vi "GoDef.vi"(8 "error in (no error)":errorcluster, 10 "String 2":string, 11 "Device in":refnum<class "Device.lvclass">) -> (0 "error out":errorcluster, 2 "String":string, 3 "Device out":refnum<class "Device.lvclass">)   [LabVIEW 2018, in "Device.lvclass"]
uses:
  Device.lvclass
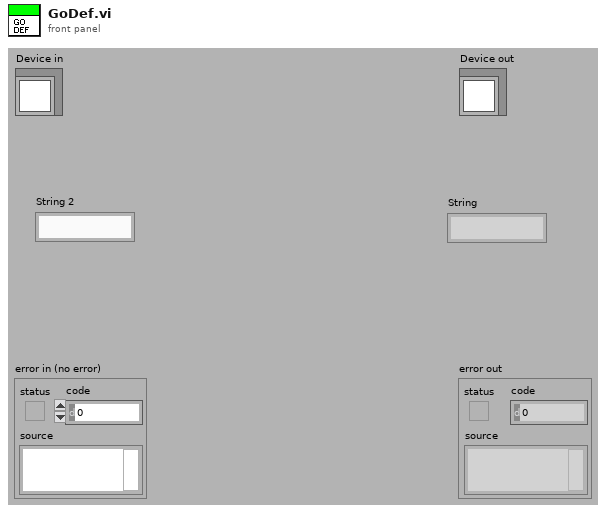
[diagram p1: front panel]
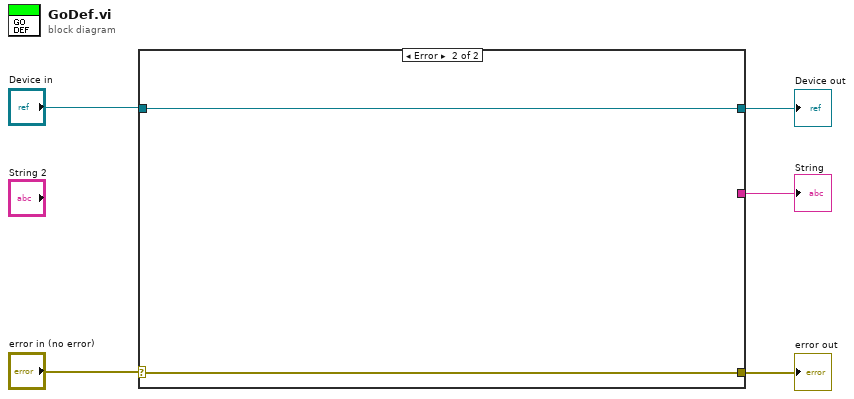
[diagram p0: block diagram]
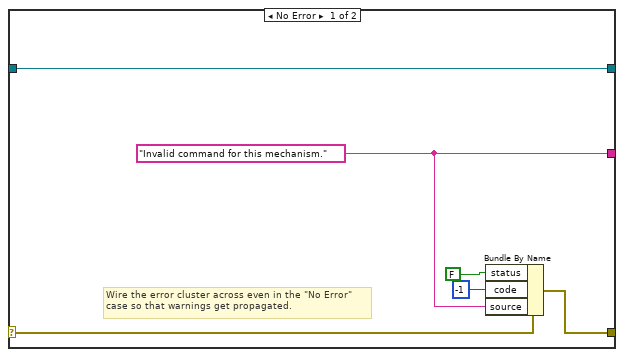
[diagram p2: hidden frame]
diagram:
  n1 = case shown="Error" "error in (no error)" {
    selector: "error in (no error)" -> [w8 w13]
    tunnel: [w7 w13] -> w2
    tunnel: [w11 w12] -> w4
    tunnel: "Device in" -> [w11 w12]
    tunnel: [w6 _] -> w3
    frame No Error {
      w6 = "Invalid command for this mechanism."
      # "Wire the error cluster across even in the \"No Error\"\ncase so that warnings get propagated."
      n2 = Bundle By Name(cluster=w8, "status"=FALSE, "code"=-1, "source"=w6) -> (w7:errorcluster)
    }
    frame Error {
    }
  }
  "error out" <- w2
  "Device out" <- w4
  "String" <- w3
